vi "Set Contact Template Variables.vi"(8 "error in (no error)":errorcluster, 9 "Index (none)":i32=-1, 10 "Contact":T1={"ID"=0, "UUID"="", "Name"="", "Iteration"=0, "Posit Array"=[], "Controls"={"throttle"=0.0, "brake"=0.0, "horn"=0.0, "wait"=0.5}, "DestArray"=[], "SetSpeed"=0.0, "Speed"=0.0}, 11 "LabVIEW Web Service Request":refnum<class "Web Request.lvclass">) -> (0 "error out":errorcluster, 3 "LabVIEW Web Service Request out":refnum<class "Web Request.lvclass">)   [LabVIEW 2014]
doc: "This VI sets all of the ESP variables for a single contact so it can be output from an ESP script."
uses:
  <vilib>/wsapi/Web Request.lvclass
  Libraries/Contact Data/Contact.ctl
  Libraries/Contact Data/Position.ctl
  Libraries/Contact Data/Controls.ctl
  Libraries/Contact Data/DestinationCluster.ctl
  Libraries/Contact Data/DesinationControls.ctl
  <vilib>/wsapi/class/subVIs/Set Many String ESP Variables.vi
  <vilib>/wsapi/class/subVIs/Set Integer ESP Variable.vi
  Libraries/Contact Data/Contact Data.lvlib
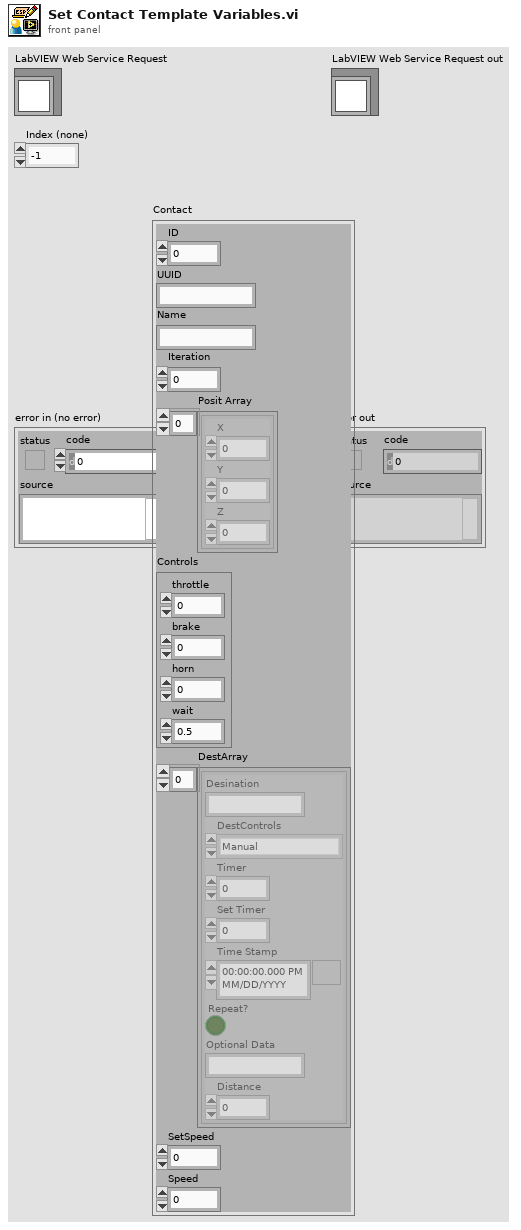
[diagram p1: front panel]
types:
  T1 = typedef "Contact Data.lvlib/Contact.ctl" = cluster{"ID":u32, "UUID":string, "Name":string, "Iteration":i32, "Posit Array":T2[], "Controls":T3, "DestArray":T4[], "SetSpeed":dbl, "Speed":dbl}
  T2 = typedef "Contact Data.lvlib/Position.ctl" = cluster{"X":dbl, "Y":dbl, "Z":dbl}
  T3 = typedef "Contact Data.lvlib/Controls.ctl" = cluster{"throttle":dbl, "brake":dbl, "horn":dbl, "wait":dbl}
  T4 = typedef "Contact Data.lvlib/DestinationCluster.ctl" = cluster{"Desination":string, "DestControls":T5, "Timer":u32, "Set Timer":u32, "Time Stamp":timestamp, "Repeat?":bool, "Optional Data":string, "Distance":dbl}
  T5 = typedef "Contact Data.lvlib/DesinationControls.ctl" = enum16{"Tracker", "Manual", "Stop", "Station DateTime", "Station Timer", "Maintain"}
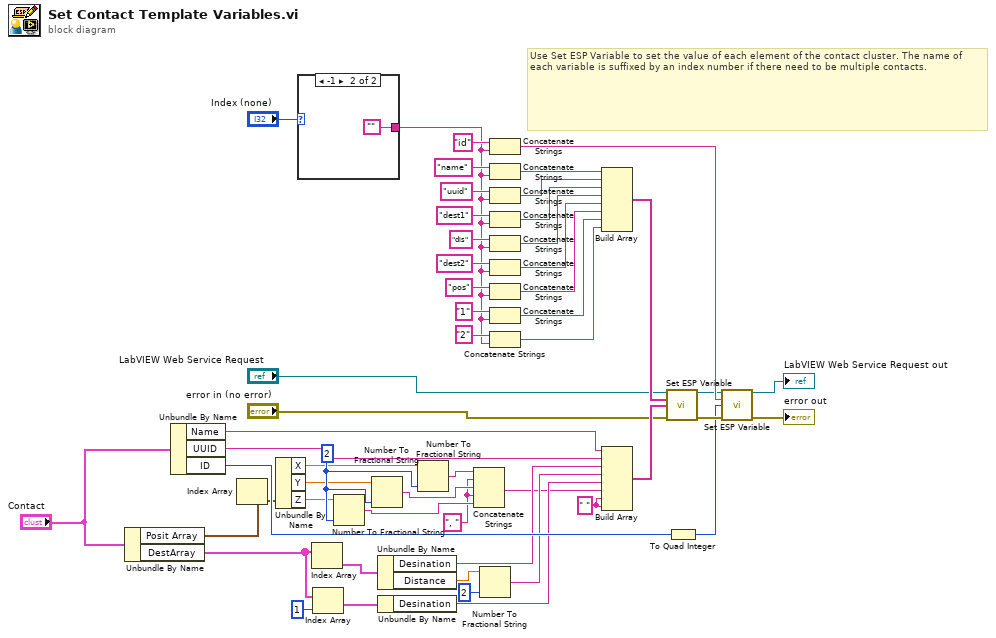
[diagram p0: block diagram]
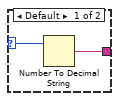
[diagram p2: hidden frame]
diagram:
  w8 = ", " ("string")
  w20 = i16 2 ("precision (6)")
  w15 = " " ("element")
  # "Use Set ESP Variable to set the value of each element of the contact cluster. The name of each variable is suffixed by an index number if there need to be multiple contacts."
  n1 = Unbundle By Name("Contact") -> ("Posit Array"=w5:T2[], "DestArray"=w19:T4[])
  n2 = Unbundle By Name("Contact") -> ("Name"=w6:string, "UUID"=w22:string, "ID"=w23:u32)
  n3 = Index Array(array=w5) -> (element=w4:T2)  [unwired: 1 in]
  n4 = Unbundle By Name(w4) -> ("X"=w3:dbl, "Y"=w2:dbl, "Z"=w1:dbl)
  n5 = case shown="-1" "Index (none)" {
    selector: "Index (none)" -> [w55 _]
    tunnel: [w56 ""] -> w42
    frame Default {
      n6 = Number To Decimal String(number=w55) -> (decimal integer string=w56:string)  [unwired: 1 in]
    }
    frame -1 {
    }
  }
  n7 = Index Array(array=w19) -> (element=w24:T4)  [unwired: 1 in]
  n8 = Index Array(array=w19, index=1) -> (element=w17:T4)
  n9 = Number To Fractional String(number=w1, precision (6)=w20) -> (F-format string=w9:string)  [unwired: 2 in]
  n10 = Number To Fractional String(number=w2, precision (6)=w20) -> (F-format string=w10:string)  [unwired: 2 in]
  n11 = Unbundle By Name(w24) -> ("Desination"=w16:string, "Distance"=w7:dbl)
  n12 = Unbundle By Name(w17) -> ("Desination"=w13:string)
  n13 = Number To Fractional String(number=w3, precision (6)=w20) -> (F-format string=w21:string)  [unwired: 2 in]
  n14 = Concatenate Strings(w21, w8, w10, w8, w9) -> (w11:string)
  n15 = Number To Fractional String(number=w7, precision (6)=i16 2) -> (F-format string=w12:string)  [unwired: 2 in]
  n16 = Concatenate Strings("id" ("string"), w42) -> (w41:string)
  n17 = Concatenate Strings("name" ("string"), w42) -> (w40:string)
  n18 = Concatenate Strings("uuid" ("string"), w42) -> (w39:string)
  n19 = Concatenate Strings("dest1" ("string"), w42) -> (w38:string)
  n20 = Concatenate Strings("dis" ("string"), w42) -> (w37:string)
  n21 = Concatenate Strings("dest2" ("string"), w42) -> (w36:string)
  n22 = Concatenate Strings("pos" ("string"), w42) -> (w35:string)
  n23 = Concatenate Strings("1" ("string"), w42) -> (w34:string)
  n24 = Concatenate Strings("2" ("string"), w42) -> (w33:string)
  n25 = Build Array(w40, w39, w38, w37, w36, w35, w34, w33) -> (w32:string[])
  n26 = Build Array(w6, w22, w16, w12, w13, w11, w15, w15) -> (w31:string[])
  n27 = call-poly <vilib>:"Set ESP Variable.vi"("LabVIEW Web Service Request"="LabVIEW Web Service Request", "keys"=w32, "values"=w31, "error in (no error)"="error in (no error)") -> ("LabVIEW Web Service Request out"=w28:refnum<class "Web Request.lvclass">, "error out"=w30:errorcluster)  [unwired: 10 in]
  n28 = To Quad Integer(1:w23) -> (0:w29:i64)
  n29 = call-poly <vilib>:"Set ESP Variable.vi"("LabVIEW Web Service Request"=w28, "key"=w41, "value"=w29, "error in (no error)"=w30) -> ("LabVIEW Web Service Request out"=→"LabVIEW Web Service Request out":refnum<class "Web Request.lvclass">, "error out"=→"error out":errorcluster)  [unwired: 10 in]
